vi "ApplyTargetConfiguration.vi"(8 "error in (no error)":errorcluster, 10 "Targets Configuration":T1, 11 ".NET Refnum in":refnum<k24>) -> (0 "error out":errorcluster, 3 ".NET Refnum out":refnum<k24>)   [LabVIEW 2017, in "VeriStandTestUtilities.lvlib"]
uses:
  VeriStandTestUtilities.lvlib
  TargetsConfiguration.ctl
  TargetPlatform.ctl
  NationalInstruments.VeriStand.SystemDefinitionAPI
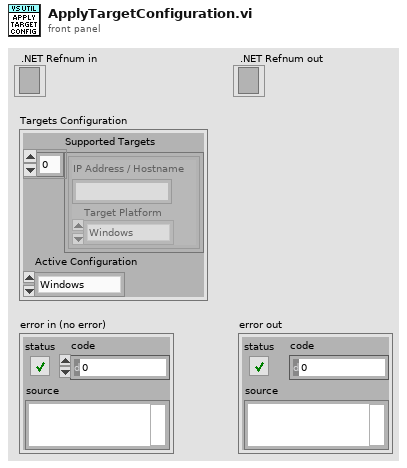
[diagram p1: front panel]
types:
  T1 = typedef "VeriStandTestUtilities.lvlib/TargetsConfiguration.ctl" = cluster{"Supported Targets":cluster{"IP Address / Hostname":string, "Target Platform":T2}[], "Active Configuration":T2}
  T2 = typedef "VeriStandTestUtilities.lvlib/TargetPlatform.ctl" = enum16{"Windows", "Linux64CRIO", "Linux64PXI", "LinuxARM", "PharLap"}
  T3 = cluster{"IP Address / Hostname":string, "Target Platform":T2}[]
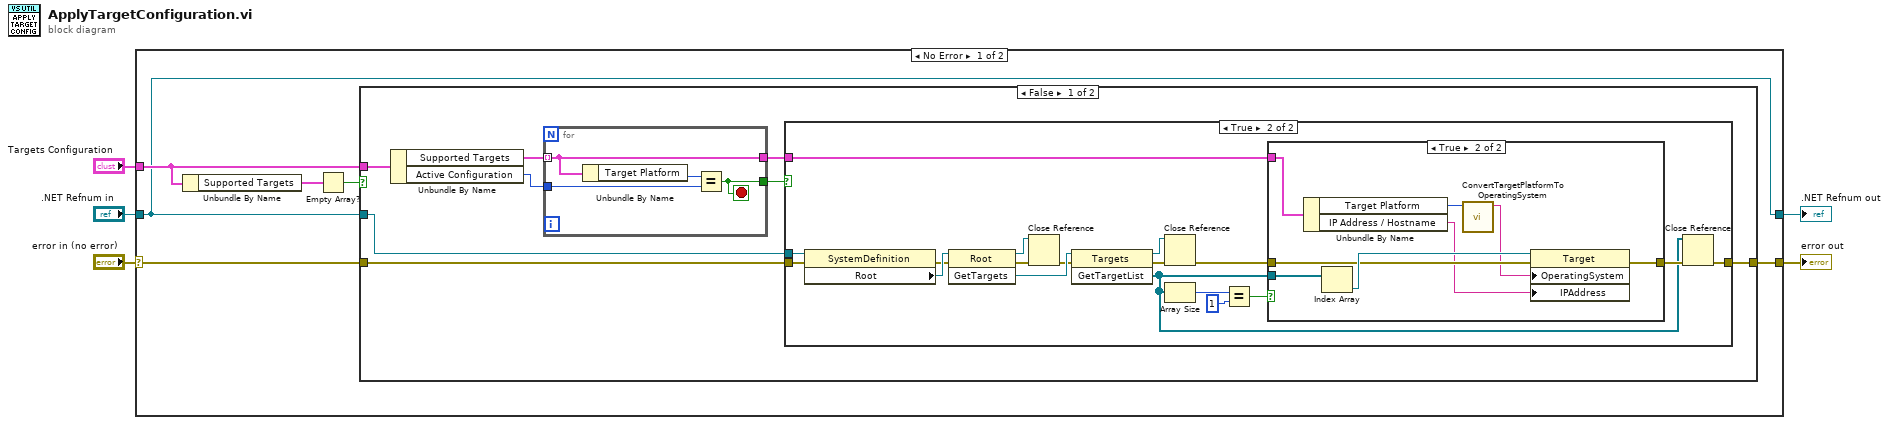
[diagram p0: block diagram]
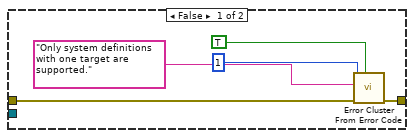
[diagram p3: hidden frame]
diagram:
  n1 = case shown="No Error" "error in (no error)" {
    selector: "error in (no error)" -> [w9 w58]
    tunnel: [w8 w58] -> w4
    tunnel: [w10 w57] -> w3
    tunnel: ".NET Refnum in" -> [w10 w57]
    tunnel: "Targets Configuration" -> [w11 _]
    frame No Error {
      n2 = Unbundle By Name(w11) -> ("Supported Targets"=w6:T3)
      n3 = Empty Array?(array=w6) -> (empty?=w7:bool)
      n4 = case shown="False" w7 {
        tunnel: w11 -> [w19 _]
        tunnel: w10 -> [w16 _]
        tunnel: w9 -> [w15 w56]
        tunnel: [w14 w56] -> w8
        frame False {
          n5 = Unbundle By Name(w19) -> ("Supported Targets"=w18:T3, "Active Configuration"=w12:T2)
          n6 = for {
            tunnel: w18 -> [w52] mode=indexing
            tunnel: w12 -> [w55]
            tunnel: [w53] -> w17
            tunnel: [w52] -> w13
            stop <- w53 stop-if-true
            n7 = Unbundle By Name(w52) -> ("Target Platform"=w54:T2)
            n8 = Equal?(x=w54, y=w55) -> (x = y?=w53:bool)
          }
          n9 = case shown="True" w17 {
            tunnel: w16 -> [_ w38]
            tunnel: w15 -> [w20 w37]
            tunnel: [w20 w23] -> w14
            tunnel: w13 -> [_ w21]
            frame False {
            }
            frame True {
              n10 = property class="SystemDefinition"(reference=w38, error in=w37) -> (error out=w28:errorcluster, "Root"=w36:refnum<k24>)  [unwired: 1 out]
              n11 = invoke class="Root" method="GetTargets"(reference=w36, error in=w28) -> (reference out=w29:refnum<k24>, error out=w31:errorcluster, "GetTargets"=w35:refnum<k24>)  [unwired: 1 in]
              n12 = Close Reference(reference=w29, error in (no error)=w31) -> (error out=w30:errorcluster)
              n13 = invoke class="Targets" method="GetTargetList"(reference=w35, error in=w30) -> (reference out=w25:refnum<k24>, error out=w27:errorcluster, "GetTargetList"=w22:refnum<k24>[])  [unwired: 1 in]
              n14 = Close Reference(reference=w25, error in (no error)=w27) -> (error out=w26:errorcluster)
              n15 = Array Size(array=w22) -> (size(s)=w34:i32)
              n16 = Equal?(x=w34, y=1) -> (x = y?=w32:bool)
              n17 = case shown="True" w32 {
                tunnel: [w43 w51] -> w24
                tunnel: w22 -> [_ w50]
                tunnel: w26 -> [w42 w48]
                tunnel: w21 -> [_ w47]
                frame False {
                  n18 = call <vilib>:"Error Cluster From Error Code.vi"("show call chain? (False)"=TRUE, "error in (no error)"=w42, "error message (\"\")"="Only system definitions with one target are supported." ("error message (\"\")"), "error code (0)"=1) -> ("error out"=w43:errorcluster)  [unwired: 5 in]
                }
                frame True {
                  n19 = Unbundle By Name(w47) -> ("Target Platform"=w45:T2, "IP Address / Hostname"=w46:string)
                  n20 = Index Array(array=w50) -> (element=w49:refnum<k24>)  [unwired: 1 in]
                  n21 = call "ConvertTargetPlatformToOperatingSystem.vi"("Platform"=w45) -> ("Operating System"=w44:string)  [unwired: 10 in]
                  n22 = property class="Target"(reference=w49, error in=w48, "OperatingSystem"=w44, "IPAddress"=w46) -> (error out=w51:errorcluster)  [unwired: 1 out]
                }
              }
              n23 = Close Reference(reference=w22, error in (no error)=w24) -> (error out=w23:errorcluster)
            }
          }
        }
        frame True {
        }
      }
    }
    frame Error {
    }
  }
  ".NET Refnum out" <- w3
  "error out" <- w4
